vi "kvCanClose.vi"(1 "error in (no error)":errorcluster, 2 "Channel Handle (input only)":i32) -> (0 "error out":errorcluster)   [LabVIEW 2023]
doc: "Closes the channel associated with the handle. If no other threads are using the circuit, it is taken off bus. The handle can not be used for further references to the channel.\n\nIf the handle is valid, then the handle is closed, regardless of input error. In this case, if there is an input error, then that error is passed to the output. If there is no input error, then the result of the close is passed to the error output.\n\nIf the handle is invalid, then the input error is passed through."
uses:
  canlib32.dll
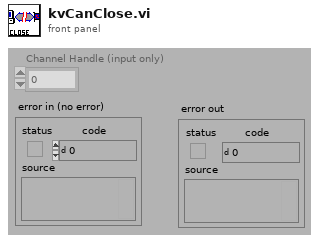
[diagram p1: front panel]
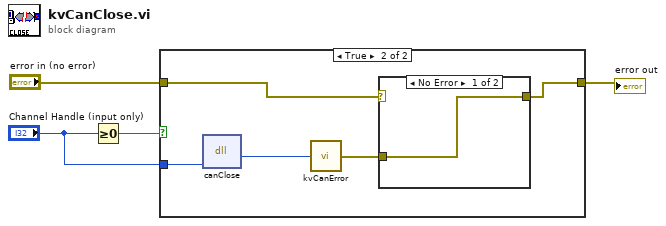
[diagram p0: block diagram]
diagram:
  n1 = Greater Or Equal To 0?(x="Channel Handle (input only)") -> (x >= 0?=w4:bool)
  n2 = case shown="True" w4 {
    tunnel: "Channel Handle (input only)" -> [_ w9]
    tunnel: "error in (no error)" -> [w5 w8]
    tunnel: [w5 w7] -> w1
    frame False {
    }
    frame True {
      n3 = dll-call lib="canlib32.dll" fn="canClose" label="Call Library Function"("channelHandle"=w9) -> (w10:i32)  [unwired: 4 in, 2 out]
      n4 = call "kvCanError.vi"("error code"=w10) -> ("error out"=w6:errorcluster)
      n5 = case shown="No Error" w8 {
        selector: w8 -> [_ w12]
        tunnel: [w11 w12] -> w7
        tunnel: w6 -> [w11 _]
        frame No Error {
        }
        frame Error {
        }
      }
    }
  }
  "error out" <- w1
